vi "PathPlanner_Trajectory_WriteCSVFile.vi"(9 "Comment":string, 10 "TRAJECTORY":T1 {"States"."TargetHolonomicRotation"."SIN" format="%13.4f"; "States"."TargetHolonomicRotation"."COS" format="%13.4f"; "States"."TargetHolonomicRotation"."VALUE" format="%13.4f"; "States"."Heading"."SIN" format="%13.4f"; "States"."Heading"."COS" format="%13.4f"; "States"."Heading"."VALUE" format="%13.4f"; "States"."PositionMeters"."Y" format="%14.3f"; "States"."PositionMeters"."X" format="%14.3f"}, 11 "FileName":string="trajectory.csv") -> (0 "error out":errorcluster)   [LabVIEW 2019, in "PathPlanner24.lvlib"]
doc: "Create a CSV file from a trajectory. This can be used on a PC or the RoboRIO. \n\nParameters:\n - FileName -- Name of the CSV file to read. See file name notes for additional information.\n - Trajectory - Trajectory data structure cluster\n - Comment - string - Optional comment to place in CSV file.\n\nReturns:\n - Error out - returned error cluster\n\nNotes on file naming:\n -- The file name must include the extention. \".csv\" is not automatically appended to the name. \n -- The file name can be a simple file or an absolute path. If a simple file name is used the default path on the RoboRIO is: \"home:\\lvuser\\natinst\\LabVIEW Data\". On a Windows PC the default path is the LabVIEW default directory. Normally this is: “%HOMEDRIVE%%HOMEPATH%\\Documents\\LabView Data\".\n -- Filenames on the RoboRIO, which runs Linux, are case sensitive.\n\nNotes on file contents:\n -- Blank lines are ignored.\n -- Lines that begin with either #, !, or ' in the first character are considered comments and are ignored. \n -- Other lines are interpretted as comma separated data"
uses:
  PathPlanner24.lvlib
  TypeDef/PathPlannerTrajectory.ctl
  TypeDef/PathPlannerTrajectoryState.ctl
  <vilib>/Rock Robotics/WPI/ThirdParty/JAS_Junk/TrajLib/TypeDef/TRANSLATION2D.ctl
  <vilib>/Rock Robotics/WPI/ThirdParty/JAS_Junk/TrajLib/TypeDef/ROTATION2D.ctl
  TypeDef/PathPlannerPathConstraints.ctl
  <vilib>/Rock Robotics/WPI/ThirdParty/JAS_Junk/TrajLib/Trajectory_Library.lvlib
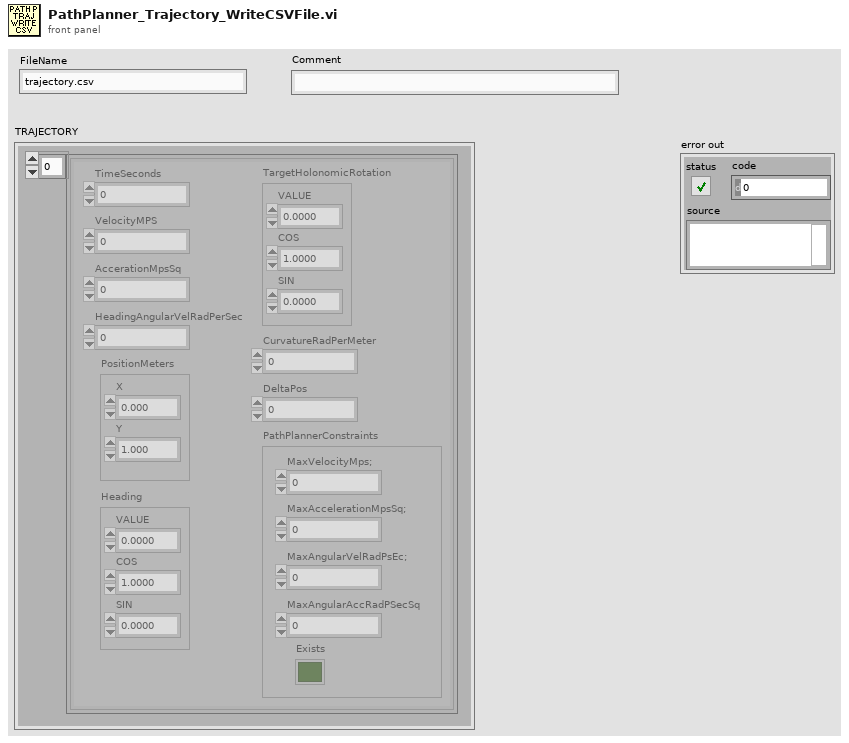
[diagram p1: front panel]
types:
  T1 = typedef "PathPlanner24.lvlib/PathPlannerTrajectory.ctl" = cluster{"States":T2[]}
  T2 = typedef "PathPlanner24.lvlib/PathPlannerTrajectoryState.ctl" = cluster{"TimeSeconds":dbl, "VelocityMPS":dbl, "AccerationMpsSq":dbl, "HeadingAngularVelRadPerSec":dbl, "PositionMeters":T3, "Heading":T4, "TargetHolonomicRotation":T4, "CurvatureRadPerMeter":dbl, "PathPlannerConstraints":T5, "DeltaPos":dbl}
  T3 = typedef "Trajectory_Library.lvlib/TRANSLATION2D.ctl" = cluster{"X":dbl, "Y":dbl}
  T4 = typedef "Trajectory_Library.lvlib/ROTATION2D.ctl" = cluster{"VALUE":dbl, "COS":dbl, "SIN":dbl}
  T5 = typedef "PathPlanner24.lvlib/PathPlannerPathConstraints.ctl" = cluster{"MaxVelocityMps;":dbl, "MaxAccelerationMpsSq;":dbl, "MaxAngularVelRadPsEc;":dbl, "MaxAngularAccRadPSecSq":dbl, "Exists":bool}
  T6 = enum16{"open", "replace", "create", "open or create", "replace or create", "replace or create with confirmation"}
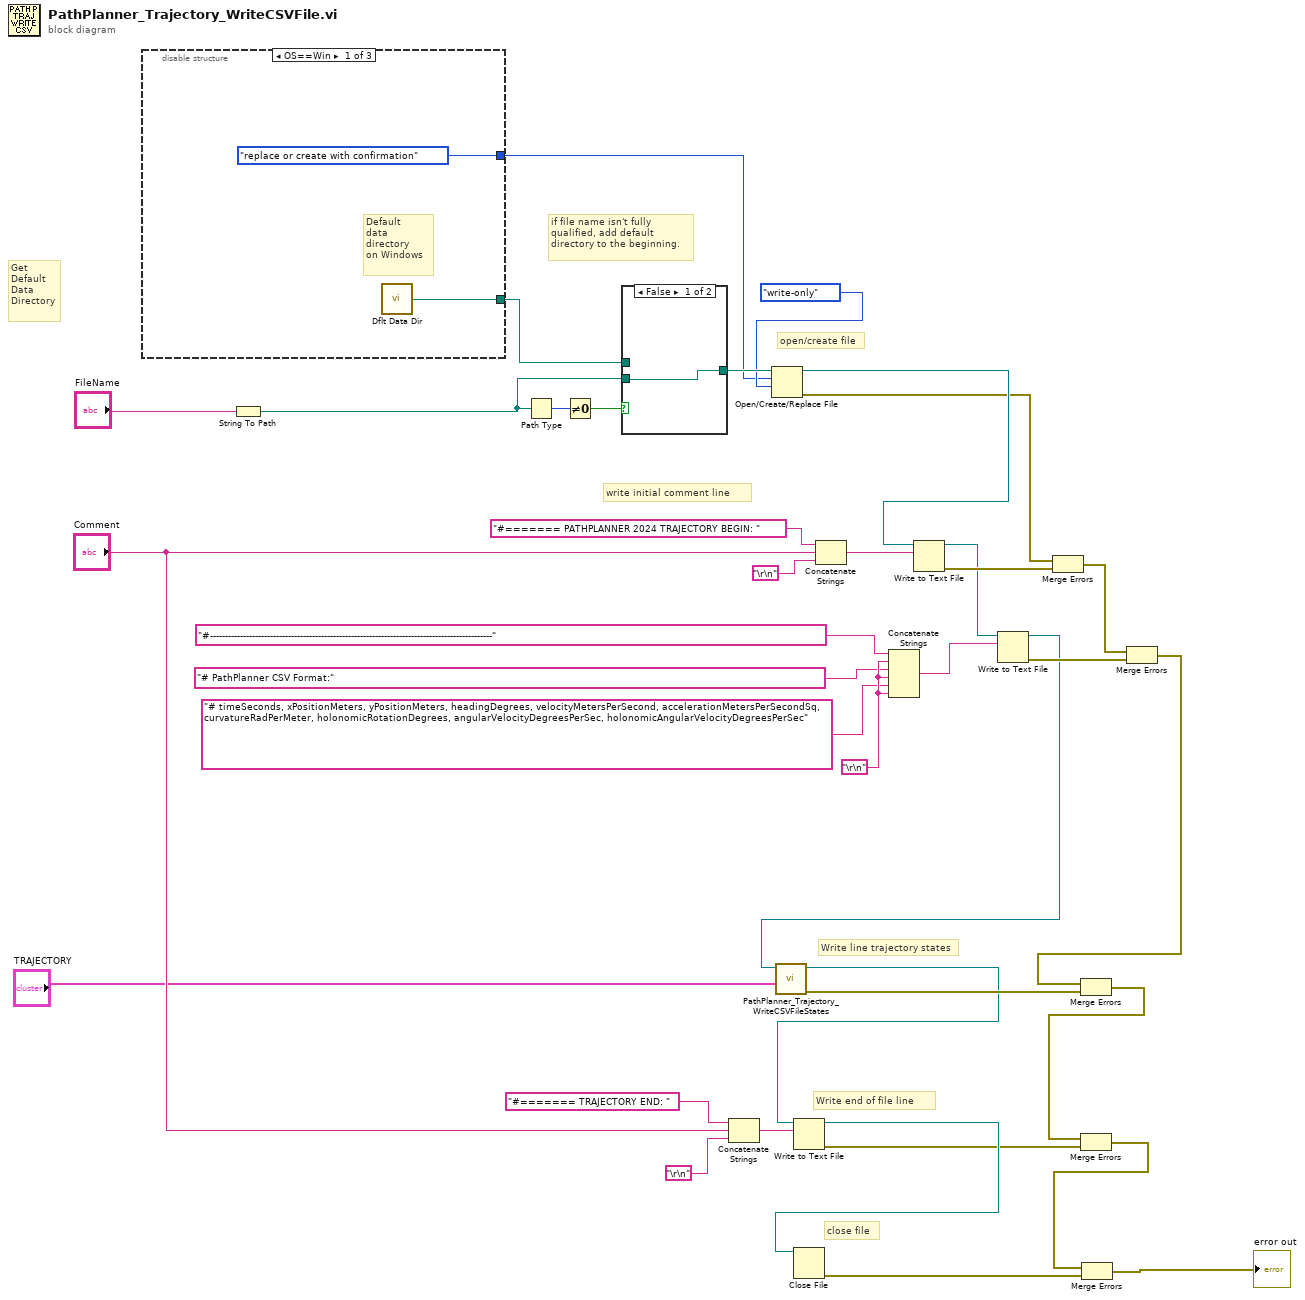
[diagram p0: block diagram]
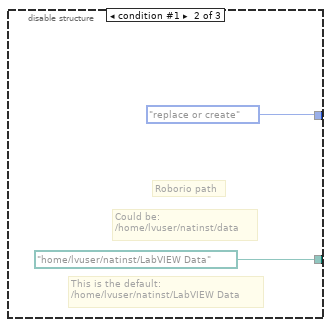
[diagram p2: hidden frame]
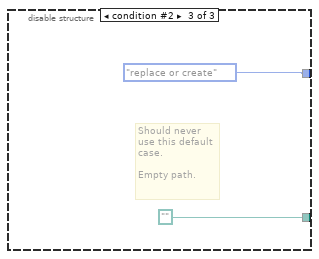
[diagram p3: hidden frame]
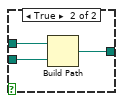
[diagram p4: hidden frame]
diagram:
  w3 = "\r\n"
  # "Write line trajectory states"
  # "open/create file"
  # "if file name isn't fully \nqualified, add default\ndirectory to the beginning."
  # "Get\nDefault\nData\nDirectory"
  # "close file"
  # "Write end of file line"
  # "write initial comment line"
  n1 = disable-structure shown="OS==Win" {
    disable-tunnel: [w39 path "/home/lvuser/natinst/LabVIEW Data" path ""] -> w28
    disable-tunnel: [T6."replace or create with confirmation" ("operation (0:open)") T6."replace or create" ("operation (0:open)") T6."replace or create" ("operation (0:open)")] -> w13
    frame condition #0 (active) {
      # "Default\ndata\ndirectory\non Windows"
      n2 = call <vilib>:"Dflt Data Dir.vi"() -> ("App:Default Data Directory"=w39:path)
    }
    frame condition #1 {
      # "This is the default:\n/home/lvuser/natinst/LabVIEW Data"
      # "Could be:\n/home/lvuser/natinst/data"
      # "Roborio path"
    }
    frame condition #2 {
      # "Should never\nuse this default\ncase.\n\nEmpty path."
    }
  }
  n3 = String To Path(string="FileName") -> (path=w4:path)
  n4 = Path Type(1:w4) -> (0:w30:i16)
  n5 = Not Equal To 0?(x=w30) -> (x != 0?=w29:bool)
  n6 = case shown="False" w29 {
    tunnel: [w44 w47] -> w27
    tunnel: w28 -> [_ w46]
    tunnel: w4 -> [w44 w45]
    frame False {
    }
    frame True {
      n7 = Build Path(base path=w46, name or relative path=w45) -> (appended path=w47:path)
    }
  }
  n8 = Concatenate Strings("#======= TRAJECTORY END: " ("string"), "Comment", "\r\n") -> (w31:string)
  n9 = Open/Create/Replace File(file path (use dialog)=w27, operation (0:open)=w13, access (0:read/write)=enum16{"read/write", "read-only", "write-only"}."write-only") -> (refnum out=w25:refnum<file>, error out=w21:errorcluster)  [unwired: 3 in, 1 out]
  n10 = Concatenate Strings("#======= PATHPLANNER 2024 TRAJECTORY BEGIN: " ("string"), "Comment", "\r\n") -> (w35:string)
  n11 = Concatenate Strings("#----------------------------------------------------------------------------------------------" ("string"), w3, "# PathPlanner CSV Format:" ("string"), w3, "# timeSeconds, xPositionMeters, yPositionMeters, headingDegrees, velocityMetersPerSecond, accelerationMetersPerSecondSq, curvatureRadPerMeter, holonomicRotationDegrees, angularVelocityDegreesPerSec, holonomicAngularVelocityDegreesPerSec" ("string"), w3) -> (w15:string)
  n12 = Write to Text File(file (use dialog)=w25, text=w35) -> (refnum out=w11:refnum<file>, error out=w22:errorcluster)  [unwired: 2 in, 1 out]
  n13 = Write to Text File(file (use dialog)=w11, text=w15) -> (refnum out=w7:refnum<file>, error out=w14:errorcluster)  [unwired: 2 in, 1 out]
  n14 = call "PathPlanner_Trajectory_WriteCSVFileStates.vi"("Trajectory"="TRAJECTORY", "Byte Steam File In"=w7) -> ("error out"=w9:errorcluster, "Byte Steam File Out"=w8:refnum<file>)  [unwired: 8 in]
  n15 = Write to Text File(file (use dialog)=w8, text=w31) -> (refnum out=w23:refnum<file>, error out=w19:errorcluster)  [unwired: 2 in, 1 out]
  n16 = Close File(refnum=w23) -> (error out=w18:errorcluster)  [unwired: 1 in, 1 out]
  n17 = Merge Errors(w21, w22) -> (w12:errorcluster)
  n18 = Merge Errors(w12, w14) -> (w10:errorcluster)
  n19 = Merge Errors(w10, w9) -> (w20:errorcluster)
  n20 = Merge Errors(w20, w19) -> (w17:errorcluster)
  n21 = Merge Errors(w17, w18) -> (→"error out":errorcluster)
